vi "Attitude Control Test1.vi"() -> ()   [LabVIEW 2022 SP3]
doc: "This example is used to make the attitude control"
uses:
  <vilib>/Utility/miscctls.llb/LV3DPointTypeDef.ctl
  lv-attitudecontrol.lvlib
panel:
  out "Boolean 3":bool
  in  "stop 4":bool
  out "Boolean 2":bool
  in  "stop 3":bool
  out "Boolean":bool
  in  "stop 2":bool
  out "Yaw":dbl
  out "Roll":dbl
  out "Pitch":dbl
  in  "Attitude Indicator":refnum<vi>(3d-picture)
  in  "stop":bool
  in  "Control 1":T1 {"X" scale=-90.0..90.0; "Y" scale=-180.0..180.0; "Z" scale=0.0..360.0}
  # "Overview: This example is used to make the attitude control\nRequirements: LabVIEW 2012 (or compatible)\nInstructions: \n1. Run this VI"
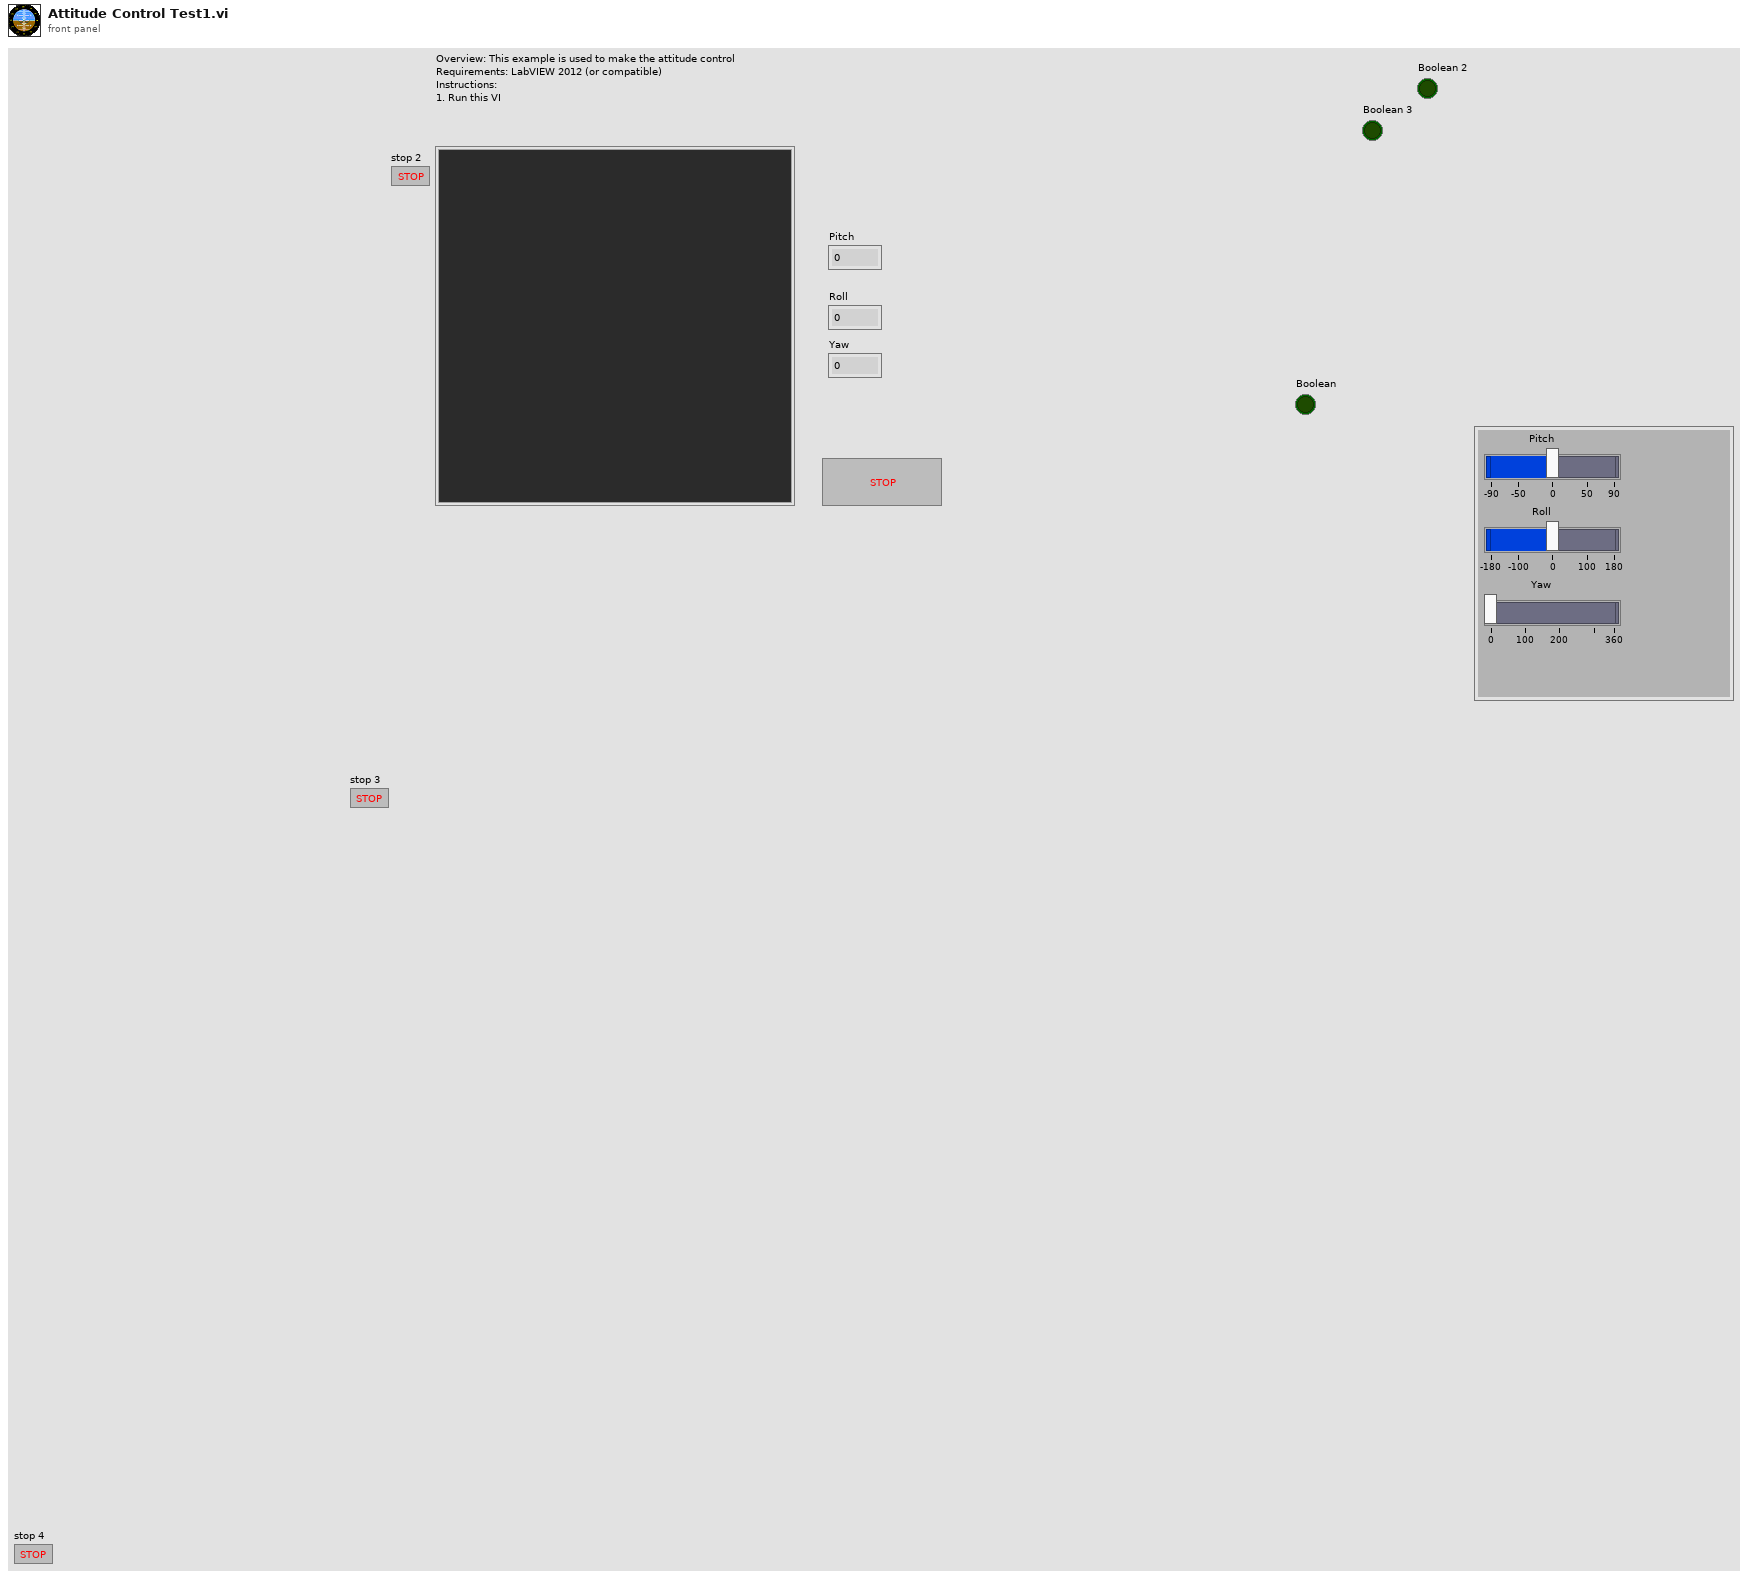
[diagram p1: front panel]
types:
  T1 = typedef "LV3DPointTypeDef.ctl" = cluster{"X":sgl, "Y":sgl, "Z":sgl}
  T2 = typedef "lv-attitudecontrol.lvlib/AttitudeHandle.ctl" = cluster{"First Scene Object":refnum<vi>, "Drum":refnum<vi>, "Window":refnum<vi>, "Dial":refnum<vi>, "Scene Graph":refnum<vi>, "Last Drum Pitch":dbl, "Last Drum Roll ":dbl, "Last Dial Roll":dbl}
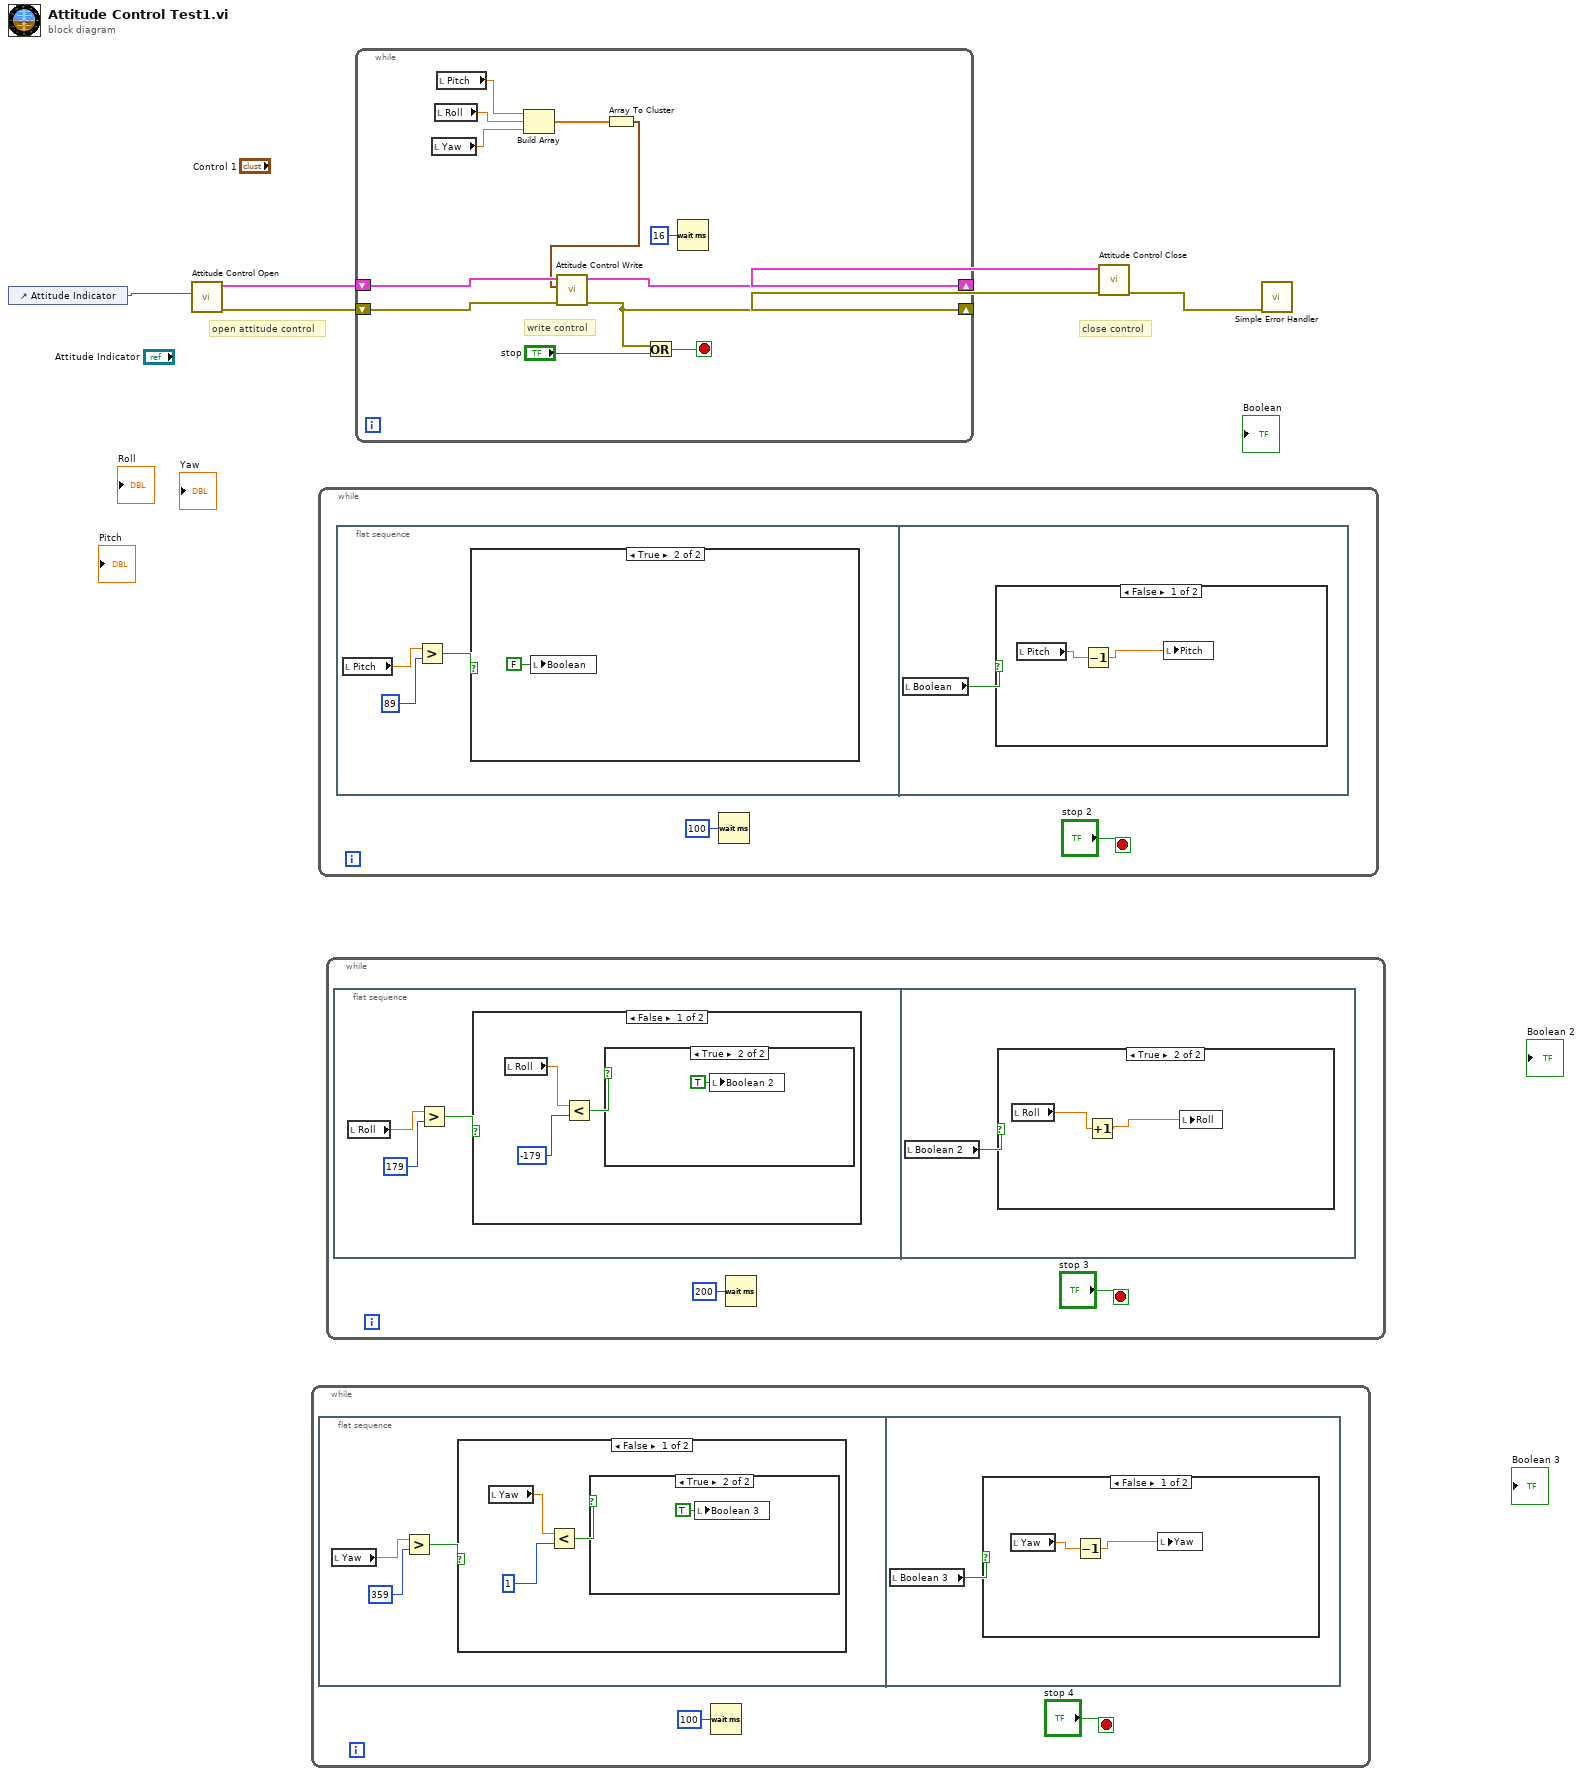
[diagram p0: block diagram]
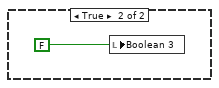
[diagram p3: hidden frame]
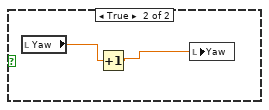
[diagram p4: hidden frame]
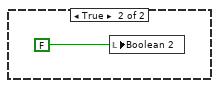
[diagram p6: hidden frame]
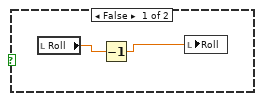
[diagram p7: hidden frame]
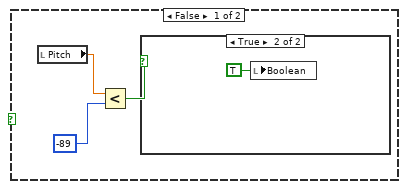
[diagram p8: hidden frame]
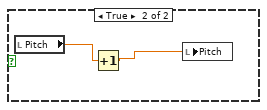
[diagram p10: hidden frame]
diagram:
  # "close control"
  # "open attitude control"
  n1 = control-ref of="Attitude Indicator"() -> (w4:refnum<vi>)
  n2 = call "Attitude Control Open.vi"("Scene Graph"=w4) -> ("error out"=w5:errorcluster, "Attitude Control Handle"=w6:T2)  [unwired: 9 in]
  n3 = while {
    stop <- "stop 4" stop-if-true
    n4 = flat-sequence {
      frame #0 {
        n5 = local read "Yaw"() -> (w11:dbl)
        n6 = Greater?(x=w11, y=359) -> (0:w9:bool)
        n7 = case shown="False" w9 {
          frame False {
            n8 = local read "Yaw"() -> (w14:dbl)
            n9 = Less?(x=w14, y=1) -> (x < y?=w12:bool)
            n10 = case shown="True" w12 {
              frame False {
              }
              frame True {
                n11 = local write "Boolean 3"(TRUE ("Boolean")) -> ()
              }
            }
          }
          frame True {
            n12 = local write "Boolean 3"(FALSE ("Boolean")) -> ()
          }
        }
      }
      frame #1 {
        n13 = local read "Boolean 3"() -> (w17:bool)
        n14 = case shown="False" w17 {
          frame False {
            n15 = local read "Yaw"() -> (w18:dbl)
            n16 = Decrement(x=w18) -> (x-1=w19:dbl)
            n17 = local write "Yaw"(w19) -> ()
          }
          frame True {
            n18 = local read "Yaw"() -> (w21:dbl)
            n19 = Increment(x=w21) -> (x+1=w20:dbl)
            n20 = local write "Yaw"(w20) -> ()
          }
        }
      }
    }
    n21 = Wait (ms)(milliseconds to wait=u32 100) -> ()  [unwired: 1 out]
  }
  n22 = while {
    stop <- "stop 2" stop-if-true
    n23 = flat-sequence {
      frame #0 {
        n24 = local read "Pitch"() -> (w26:dbl)
        n25 = Greater?(x=w26, y=89) -> (0:w24:bool)
        n26 = case shown="True" w24 {
          frame False {
            n27 = local read "Pitch"() -> (w29:dbl)
            n28 = Less?(x=w29, y=-89) -> (x < y?=w27:bool)
            n29 = case shown="True" w27 {
              frame False {
              }
              frame True {
                n30 = local write "Boolean"(TRUE ("Boolean")) -> ()
              }
            }
          }
          frame True {
            n31 = local write "Boolean"(FALSE ("Boolean")) -> ()
          }
        }
      }
      frame #1 {
        n32 = local read "Boolean"() -> (w32:bool)
        n33 = case shown="False" w32 {
          frame False {
            n34 = local read "Pitch"() -> (w33:dbl)
            n35 = Decrement(x=w33) -> (x-1=w34:dbl)
            n36 = local write "Pitch"(w34) -> ()
          }
          frame True {
            n37 = local read "Pitch"() -> (w36:dbl)
            n38 = Increment(x=w36) -> (x+1=w35:dbl)
            n39 = local write "Pitch"(w35) -> ()
          }
        }
      }
    }
    n40 = Wait (ms)(milliseconds to wait=u32 100) -> ()  [unwired: 1 out]
  }
  n41 = while {
    stop <- "stop 3" stop-if-true
    n42 = flat-sequence {
      frame #0 {
        n43 = local read "Roll"() -> (w41:dbl)
        n44 = Greater?(x=w41, y=179) -> (0:w39:bool)
        n45 = case shown="False" w39 {
          frame False {
            n46 = local read "Roll"() -> (w44:dbl)
            n47 = Less?(x=w44, y=-179) -> (x < y?=w42:bool)
            n48 = case shown="True" w42 {
              frame False {
              }
              frame True {
                n49 = local write "Boolean 2"(TRUE ("Boolean")) -> ()
              }
            }
          }
          frame True {
            n50 = local write "Boolean 2"(FALSE ("Boolean")) -> ()
          }
        }
      }
      frame #1 {
        n51 = local read "Boolean 2"() -> (w47:bool)
        n52 = case shown="True" w47 {
          frame False {
            n53 = local read "Roll"() -> (w48:dbl)
            n54 = Decrement(x=w48) -> (x-1=w49:dbl)
            n55 = local write "Roll"(w49) -> ()
          }
          frame True {
            n56 = local read "Roll"() -> (w51:dbl)
            n57 = Increment(x=w51) -> (x+1=w50:dbl)
            n58 = local write "Roll"(w50) -> ()
          }
        }
      }
    }
    n59 = Wait (ms)(milliseconds to wait=u32 200) -> ()  [unwired: 1 out]
  }
  n60 = while {
    shift-right: [w57] -> w2
    shift-left: w6 -> [w63]
    shift-right: [w58] -> w3
    shift-left: w5 -> [w62]
    stop <- w59 stop-if-true
    # "write control"
    n61 = local read "Yaw"() -> (w54:dbl)
    n62 = local read "Roll"() -> (w55:dbl)
    n63 = local read "Pitch"() -> (w56:dbl)
    n64 = Build Array(w56, w55, w54) -> (w53:dbl[])
    n65 = Array To Cluster(array=w53) -> (cluster=w52:cluster{"[0]":dbl, "[1]":dbl, "[2]":dbl})
    n66 = call "Attitude Control Write.vi"("error in (no error)"=w62, "pitch (x), roll (y), yaw (z)"=w52, "Attitude Control Handle In"=w63) -> ("error out"=w58:errorcluster, "Attitude Control Handle Out"=w57:T2)  [unwired: 7 in]
    n67 = Or(x=w58, y="stop") -> (x .or. y?=w59:bool)
    n68 = Wait (ms)(milliseconds to wait=u32 16) -> ()  [unwired: 1 out]
  }
  n69 = call "Attitude Control Close.vi"("error in (no error)"=w3, "Attitude Control Handle"=w2) -> ("error out"=w1:errorcluster)  [unwired: 9 in]
  n70 = call <vilib>:"Simple Error Handler.vi"("error in (no error)"=w1) -> ()  [unwired: 4 in, 5 out]
